vi "m1m3_getEvent_ForceActuatorInfo.vi"(8 "error in (no error)":errorcluster, 11 "logevent_ForceActuatorInfo_Ctl":T1) -> (0 "error out":errorcluster, 2 "function return":i32, 3 "logevent_ForceActuatorInfo_Ctl out":T1)   [LabVIEW 2016, in "SALLV_m1m3.lvlib"]
doc: "int m1m3_shm_getEvent_ForceActuatorInfoLV(m1m3_logevent_ForceActuatorInfoLV *logevent_ForceActuatorInfo_Ctl );"
uses:
  SALLV_m1m3.lvlib
  DataTypes/logevent_ForceActuatorInfo.ctl
  SALLV_m1m3.so
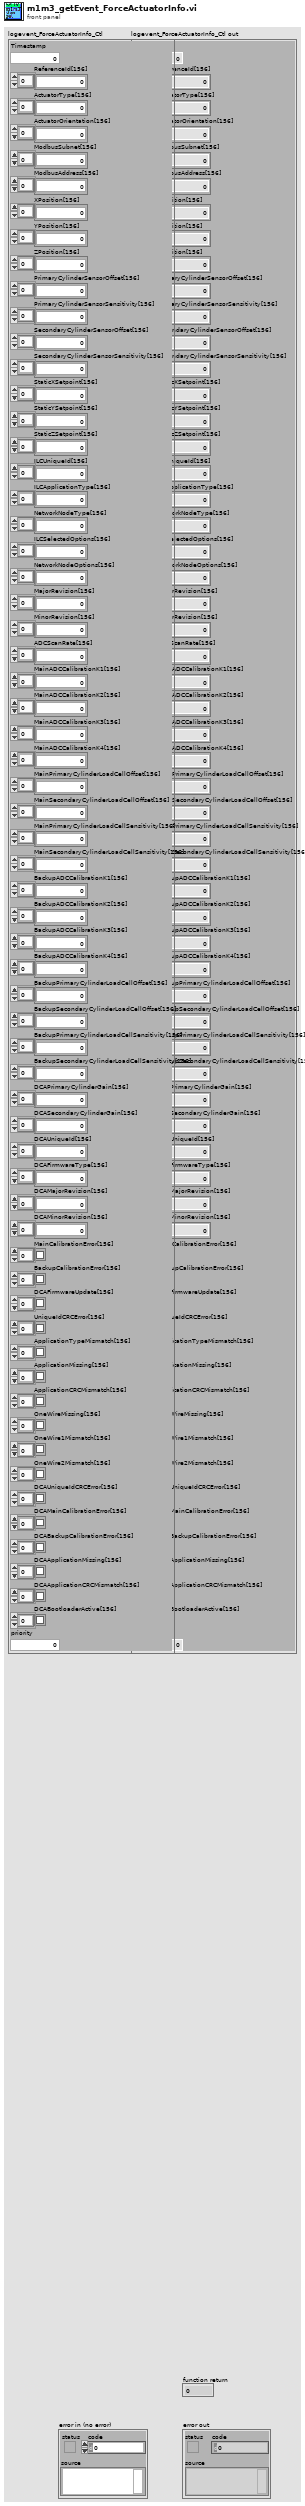
[diagram p1: front panel]
types:
  T1 = typedef "SALLV_m1m3.lvlib/logevent_ForceActuatorInfo.ctl" = cluster{"Timestamp":dbl, "ReferenceId[156]":i32[], "ActuatorType[156]":i32[], "ActuatorOrientation[156]":i32[], "ModbusSubnet[156]":u8[], "ModbusAddress[156]":u8[], "XPosition[156]":sgl[], "YPosition[156]":sgl[], "ZPosition[156]":sgl[], "PrimaryCylinderSensorOffset[156]":sgl[], "PrimaryCylinderSensorSensitivity[156]":sgl[], "SecondaryCylinderSensorOffset[156]":sgl[], "SecondaryCylinderSensorSensitivity[156]":sgl[], "StaticXSetpoint[156]":dbl[], "StaticYSetpoint[156]":dbl[], "StaticZSetpoint[156]":dbl[], "ILCUniqueId[156]":i64[], "ILCApplicationType[156]":u8[], "NetworkNodeType[156]":u8[], "ILCSelectedOptions[156]":u8[], "NetworkNodeOptions[156]":u8[], "MajorRevision[156]":u8[], "MinorRevision[156]":u8[], "ADCScanRate[156]":u8[], "MainADCCalibrationK1[156]":sgl[], "MainADCCalibrationK2[156]":sgl[], "MainADCCalibrationK3[156]":sgl[], "MainADCCalibrationK4[156]":sgl[], "MainPrimaryCylinderLoadCellOffset[156]":sgl[], "MainSecondaryCylinderLoadCellOffset[156]":sgl[], "MainPrimaryCylinderLoadCellSensitivity[156]":sgl[], "MainSecondaryCylinderLoadCellSensitivity[156]":sgl[], "BackupADCCalibrationK1[156]":sgl[], "BackupADCCalibrationK2[156]":sgl[], "BackupADCCalibrationK3[156]":sgl[], "BackupADCCalibrationK4[156]":sgl[], "BackupPrimaryCylinderLoadCellOffset[156]":sgl[], "BackupSecondaryCylinderLoadCellOffset[156]":sgl[], "BackupPrimaryCylinderLoadCellSensitivity[156]":sgl[], "BackupSecondaryCylinderLoadCellSensitivity[156]":sgl[], "DCAPrimaryCylinderGain[156]":sgl[], "DCASecondaryCylinderGain[156]":sgl[], "DCAUniqueId[156]":i64[], "DCAFirmwareType[156]":u8[], "DCAMajorRevision[156]":u8[], "DCAMinorRevision[156]":u8[], "MainCalibrationError[156]":bool[], "BackupCalibrationError[156]":bool[], "DCAFirmwareUpdate[156]":bool[], "UniqueIdCRCError[156]":bool[], "ApplicationTypeMismatch[156]":bool[], "ApplicationMissing[156]":bool[], "ApplicationCRCMismatch[156]":bool[], "OneWireMissing[156]":bool[], "OneWire1Mismatch[156]":bool[], "OneWire2Mismatch[156]":bool[], "DCAUniqueIdCRCError[156]":bool[], "DCAMainCalibrationError[156]":bool[], "DCABackupCalibrationError[156]":bool[], "DCAApplicationMissing[156]":bool[], "DCAApplicationCRCMismatch[156]":bool[], "DCABootloaderActive[156]":bool[], "priority":i32}
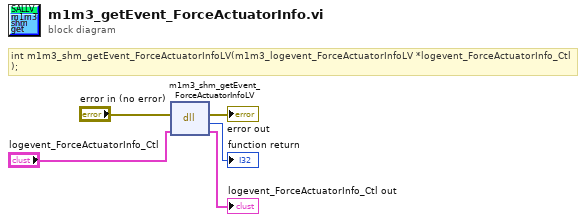
[diagram p0: block diagram]
diagram:
  # "int m1m3_shm_getEvent_ForceActuatorInfoLV(m1m3_logevent_ForceActuatorInfoLV *logevent_ForceActuatorInfo_Ctl );"
  n1 = dll-call lib="opt/CODE/SALLV_m1m3/SALLV_m1m3.*" fn="m1m3_shm_getEvent_ForceActuatorInfoLV"(error in="error in (no error)", "logevent_ForceActuatorInfo_Ctl"="logevent_ForceActuatorInfo_Ctl") -> (error out=→"error out":errorcluster, →"function return":i32, "logevent_ForceActuatorInfo_Ctl"=→"logevent_ForceActuatorInfo_Ctl out":T1)  [unwired: 2 in, 1 out]
